vi "To Local Coordinates.vi"(8 "error in":errorcluster, 10 "Center/Orientation":T1, 11 "Global Coordinates":refnum<class "Vec3d Class.lvclass">) -> (0 "error out":errorcluster, 3 "Local Coordinates":refnum<class "Vec3d Class.lvclass">)   [LabVIEW 2011]
uses:
  Type Definitions/Position_Orientation.ctl
  Vec3d Class/Vec3d Class.lvclass
  Orient3d Class/Orient3d Class.lvclass
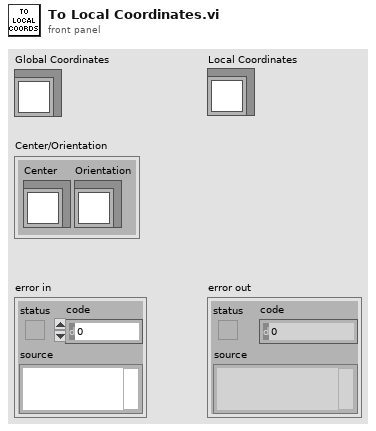
[diagram p1: front panel]
types:
  T1 = typedef "Position_Orientation.ctl" = cluster{"Center":refnum<class "Vec3d Class.lvclass">, "Orientation":refnum<class "Orient3d Class.lvclass">}
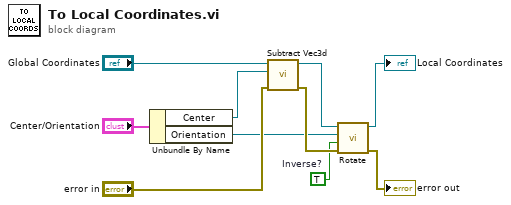
[diagram p0: block diagram]
diagram:
  w1 = TRUE  # Inverse?
  n1 = Unbundle By Name("Center/Orientation") -> ("Center"=w8:refnum<class "Vec3d Class.lvclass">, "Orientation"=w2:refnum<class "Orient3d Class.lvclass">)
  n2 = call "Subtract Vec3d.vi"("error in (no error)"="error in", "Vec3d in 2"=w8, "Vec3d in 1"="Global Coordinates") -> ("error out"=w4:errorcluster, "Vec3d Class out"=w6:refnum<class "Vec3d Class.lvclass">)  [unwired: 7 in]
  n3 = call-dynamic "Rotate.vi"("error in"=w4, "Inverse?"=w1, "Orient3d in"=w2, "Vec3d in"=w6) -> ("error out"=→"error out":errorcluster, "Vec3d out"=→"Local Coordinates":refnum<class "Vec3d Class.lvclass">)  [unwired: 6 in]
